vi "左转0.85？.vi"(0 "PWM1":T8, 1 "PWM 2":T8, 2 "PWM 3":T8, 3 "PWM 4":T8, 4 "DIO":T1, 5 "错误输入":errorcluster, 6 "当前角度":dbl, 7 "目标角度":dbl) -> (8 "错误输出":errorcluster)   [LabVIEW 2016]
uses:
  <vilib>/myRIO/Instrument Drivers/Onboard IO/PWM/typedefs/PWM Reference.ctl
  <vilib>/myRIO/Common/Instrument Driver Framework/Utilities/typedefs/myRIO Generic Hardware Reference.ctl
  <vilib>/myRIO/Common/Instrument Driver Framework/Utilities/typedefs/Hardware Version Enum.ctl
  <vilib>/myRIO/Common/Instrument Driver Framework/Utilities/typedefs/myRIO v1.0 Reference.ctl
  <vilib>/myRIO/Common/Instrument Driver Framework/Utilities/typedefs/Generic FPGA Reference.ctl
  <vilib>/myRIO/Common/Instrument Driver Framework/myRIO v1.0/PWM/typedefs/PWM Channels Enum.ctl
  <vilib>/myRIO/Instrument Drivers/Onboard IO/PWM/typedefs/PWM Configuration.ctl
  <vilib>/myRIO/Instrument Drivers/Onboard IO/DIO/typedefs/DIO Reference.ctl
  <vilib>/myRIO/Common/Instrument Driver Framework/myRIO v1.0/DIO/typedefs/DIO Channels List.ctl
  <vilib>/myRIO/Common/Instrument Driver Framework/myRIO v1.0/DIO/typedefs/DIO Channels Enum.ctl
  <vilib>/myRIO/Instrument Drivers/Onboard IO/PWM/PWM.lvlib
  <vilib>/myRIO/Instrument Drivers/Onboard IO/DIO/DIO.lvlib
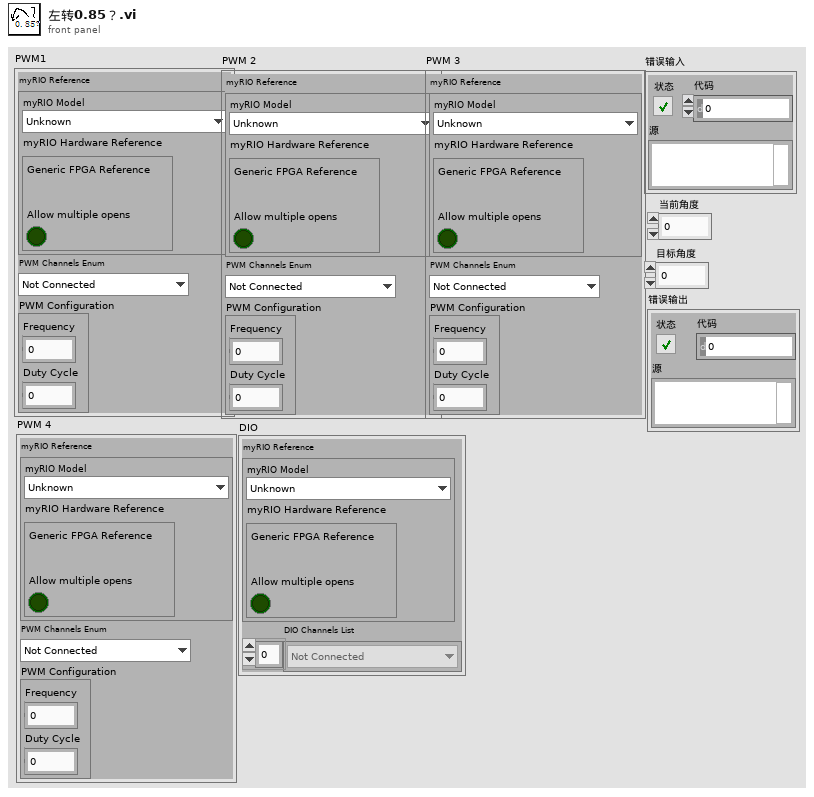
[diagram p1: front panel]
types:
  T1 = typedef "DIO.lvlib/DIO Reference.ctl" = cluster{"myRIO Reference":T2, "DIO Channels List":T6}
  T2 = typedef "myRIO Generic Hardware Reference.ctl" = cluster{"myRIO Model":T3, "myRIO Hardware Reference":T4}
  T3 = typedef "Hardware Version Enum.ctl" = enum16{"Unknown", "myRIO-1900", "myRIO-1950", "roboRIO", "NI ELVIS RIO CM"}
  T4 = typedef "myRIO v1.0 Reference.ctl" = cluster{"Generic FPGA Reference":T5, "Allow multiple opens":bool}
  T5 = typedef "Generic FPGA Reference.ctl" = refnum<k20>
  T6 = typedef "DIO Channels List.ctl" = T7[]
  T7 = typedef "DIO Channels Enum.ctl" = enum16{"Not Connected", "C/DIO0", "C/DIO1", "C/DIO2", "C/DIO3", "C/DIO4", "C/DIO5", "C/DIO6", "C/DIO7", "A/DIO0", "A/DIO1", "A/DIO2", "A/DIO3", "A/DIO4", "A/DIO5", "A/DIO6", "A/DIO7", "A/DIO8", "A/DIO9", "A/DIO10", "A/DIO11", "A/DIO12", "A/DIO13", "A/DIO14", "A/DIO15", "B/DIO0", "B/DIO1", "B/DIO2", "B/DIO3", "B/DIO4", "B/DIO5", "B/DIO6", "B/DIO7", "B/DIO8", "B/DIO9", "B/DIO10", "B/DIO11", "B/DIO12", "B/DIO13", "B/DIO14", "B/DIO15", "LED0", "LED1", "LED2", "LED3", "Button0", "DIO/DIO0", "DIO/DIO1", "DIO/DIO2", "DIO/DIO3", "DIO/DIO4", "DIO/DIO5", "DIO/DIO6", "DIO/DIO7", "DIO/DIO8", "DIO/DIO9", "SPI/CS0", "SPI/CS1", "SPI/CS2", "SPI/CS3", "LED RADIO (Green)", "LED RADIO (Red)", "LED COMM (Green)", "LED COMM (Red)", "LED MODE (Green)", "LED MODE (Red)"}
  T8 = typedef "PWM.lvlib/PWM Reference.ctl" = cluster{"myRIO Reference":T2, "PWM Channels Enum":T9, "PWM Configuration":T10}
  T9 = typedef "PWM Channels Enum.ctl" = enum16{"Not Connected", "C/PWM0", "C/PWM1", "A/PWM0", "A/PWM1", "A/PWM2", "B/PWM0", "B/PWM1", "B/PWM2", "PWM/PWM0", "PWM/PWM1", "PWM/PWM2", "PWM/PWM3", "PWM/PWM4", "PWM/PWM5", "PWM/PWM6", "PWM/PWM7", "PWM/PWM8", "PWM/PWM9"}
  T10 = typedef "PWM.lvlib/PWM Configuration.ctl" = cluster{"Frequency":dbl, "Duty Cycle":dbl}
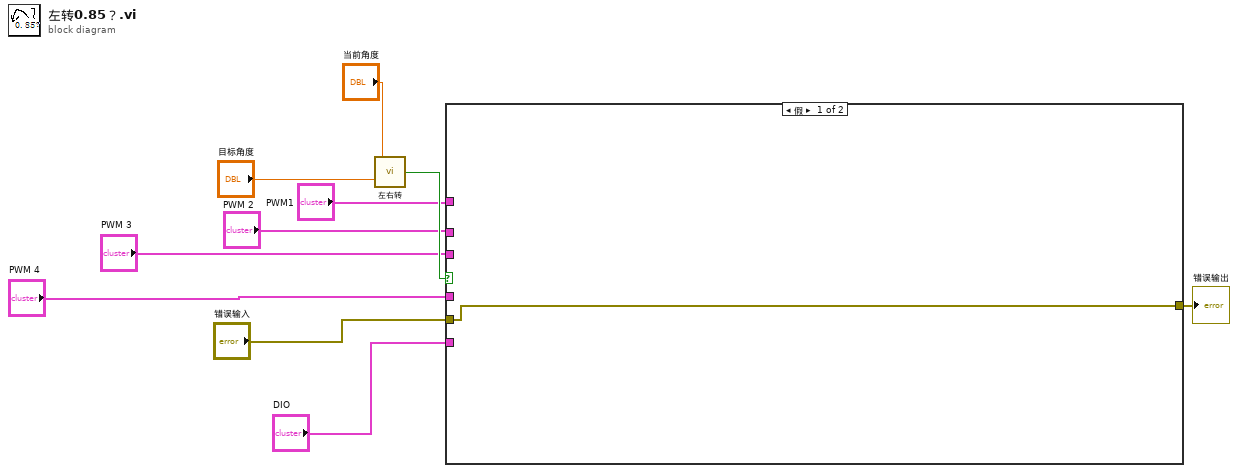
[diagram p0: block diagram]
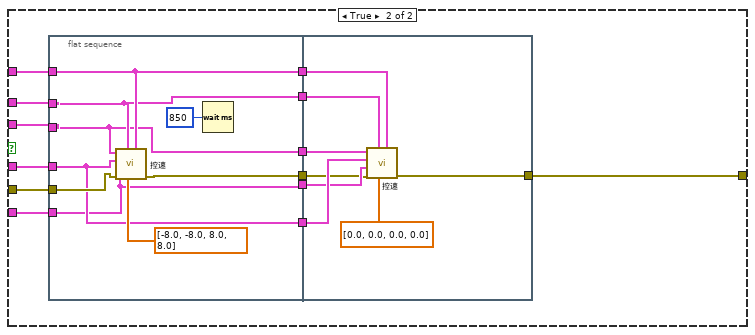
[diagram p2: hidden frame]
diagram:
  n1 = call "左右转.vi"("目标角度"="目标角度", "当前角度"="当前角度") -> ("左转/右转"=w10:bool)
  n2 = case shown="假" w10 {
    tunnel: "错误输入" -> [w11 w24]
    tunnel: "PWM1" -> [_ w23]
    tunnel: "PWM 2" -> [_ w22]
    tunnel: "PWM 3" -> [_ w21]
    tunnel: "PWM 4" -> [_ w20]
    tunnel: "DIO" -> [_ w19]
    tunnel: [w11 w12] -> w1
    frame False {
    }
    frame True {
      n3 = flat-sequence {
        tunnel: w24 -> [w33]
        tunnel: w23 -> [w30]
        tunnel: w22 -> [w29]
        tunnel: w21 -> [w28]
        tunnel: w20 -> [w27]
        tunnel: w19 -> [w26]
        tunnel: [w30] -> w18
        tunnel: [w29] -> w17
        tunnel: [w28] -> w16
        tunnel: [w27] -> w15
        tunnel: [w26] -> w14
        tunnel: [w25] -> w13
        tunnel: w18 -> [w41]
        tunnel: w17 -> [w40]
        tunnel: w16 -> [w39]
        tunnel: w15 -> [w38]
        tunnel: w14 -> [w37]
        tunnel: w13 -> [w36]
        tunnel: [w34] -> w12
        frame #0 {
          n4 = call "控速.vi"("PWM1"=w30, "速度"=dbl[] [-8.0, -8.0, 8.0, 8.0], "PWM2"=w29, "错误输入（无错误）"=w33, "DIO"=w26, "PWM 4"=w27, "PWM 3"=w28) -> ("错误输出"=w25:errorcluster)  [unwired: 4 in]
          n5 = Wait (ms)(milliseconds to wait=u32 850 ("等待时间（毫秒）")) -> ()  [unwired: 1 out]
        }
        frame #1 {
          n6 = call "控速.vi"("PWM1"=w41, "速度"=dbl[] [0.0, 0.0, 0.0, 0.0], "PWM2"=w40, "错误输入（无错误）"=w36, "DIO"=w37, "PWM 4"=w38, "PWM 3"=w39) -> ("错误输出"=w34:errorcluster)  [unwired: 4 in]
        }
      }
    }
  }
  "错误输出" <- w1
